vi "TreeUpdate.vi"(8 "error in":errorcluster, 11 "Data input":T1) -> (0 "error out":errorcluster, 3 "Data output":T1)   [LabVIEW 2017]
doc: "<B>This VI is used for updating tree item with Caps properties.</B>"
uses:
  API/Tree/SLSC Tree Control.lvlib
  Ctrl/Property.ctl
  Ctrl/PhysicalChannel.ctl
  Ctrl/Bitfield.ctl
  Ctrl/Register.ctl
  Ctrl/ScaleType.ctl
  Ctrl/Scale.ctl
  Ctrl/EnumValue.ctl
  Ctrl/Enum.ctl
  Ctrl/Caps.ctl
  Ctrl/Data.ctl
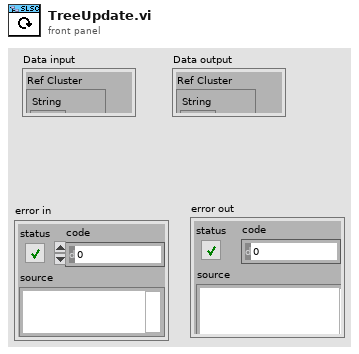
[diagram p1: front panel]
types:
  T1 = typedef "Data.ctl" = cluster{"Ref Cluster":cluster{"String":refnum<vi>, "U8":refnum<vi>, "I8":refnum<vi>, "U32":refnum<vi>, "I32":refnum<vi>, "U64":refnum<vi>, "I64":refnum<vi>, "Ring":refnum<vi>, "DBL":refnum<vi>, "Add":refnum<vi>, "Remove":refnum<vi>, "Property tree":refnum<vi>, "confirm":refnum<vi>}, "JSON Text":string, "Original JSON Text":string, "Caps":T2, "SLSC Output Tree":cluster{"Left Cell String":string, "Child Text":string[], "Child Tag":string, "Item Indent":i32, "Child Only?":bool, "Glyph Index":i32, "offline value":variant}[], "Ref Index and Control Type":cluster{"index":i32, "Datatype":string}, "Selected Type and name":cluster{"Selected Type":enum16{"Property", "Physical Channel", "Other"}, "Selected Property Name":string}, "Update whole Tree?":bool}
  T2 = typedef "Caps.ctl" = cluster{"properties":T3[], "physical channels":T4[], "registers":T5[], "scales":T7[], "enums":T9[], "productName":string}
  T3 = typedef "Property.ctl" = cluster{"name":string, "bitfield":string, "value":variant, "dataType":string, "min":variant, "max":variant, "scale":string, "access":string}
  T4 = typedef "PhysicalChannel.ctl" = cluster{"name":string, "properties":T3[]}
  T5 = typedef "Register.ctl" = cluster{"name":string, "address":i32, "size":i32, "bitfields":T6[], "initialValue":variant, "connectedProperties":string[]}
  T6 = typedef "Bitfield.ctl" = cluster{"name":string, "offset":i32, "size":i32, "signed":bool}
  T7 = typedef "Scale.ctl" = cluster{"name":string, "type":T8, "params":variant}
  T8 = typedef "ScaleType.ctl" = enum16{"NoScale", "Table", "Polynomial", "Linear"}
  T9 = typedef "Enum.ctl" = cluster{"name":string, "values":T10[]}
  T10 = typedef "EnumValue.ctl" = cluster{"name":string, "value":i32}
  T11 = cluster{"name":string, "string enums":string, "values":T10[]}[]
  T12 = cluster{"Left Cell String":string, "Child Text":string[], "Child Tag":string, "Item Indent":i32, "Child Only?":bool, "Glyph Index":i32, "offline value":variant}[]
  T13 = cluster{"Left Cell String":string, "Child Text":string[], "Child Tag":string, "Item Indent":i32, "Child Only?":bool, "Glyph Index":i32, "offline value":variant}
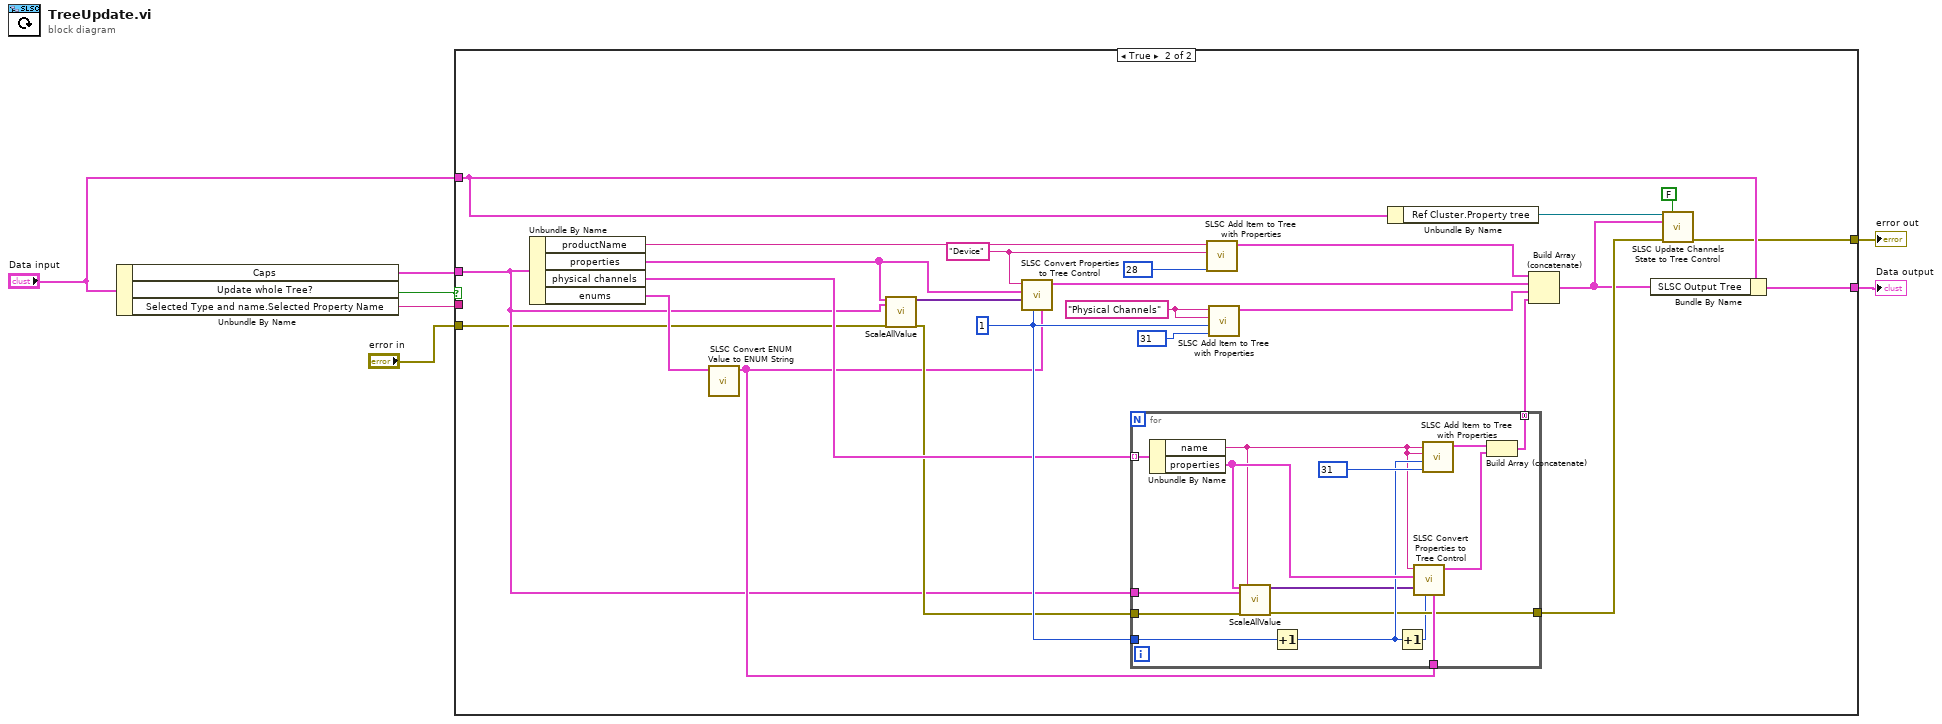
[diagram p0: block diagram]
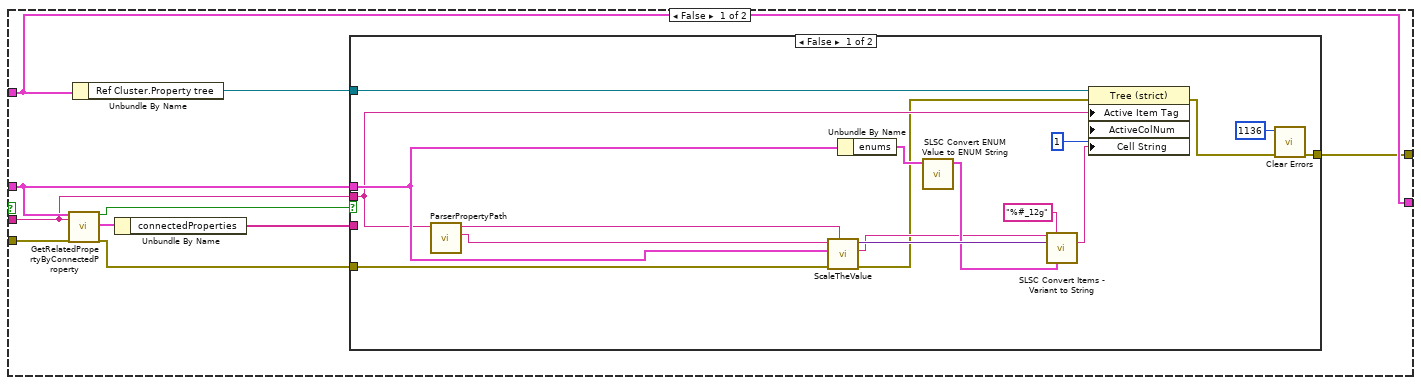
[diagram p2: hidden frame]
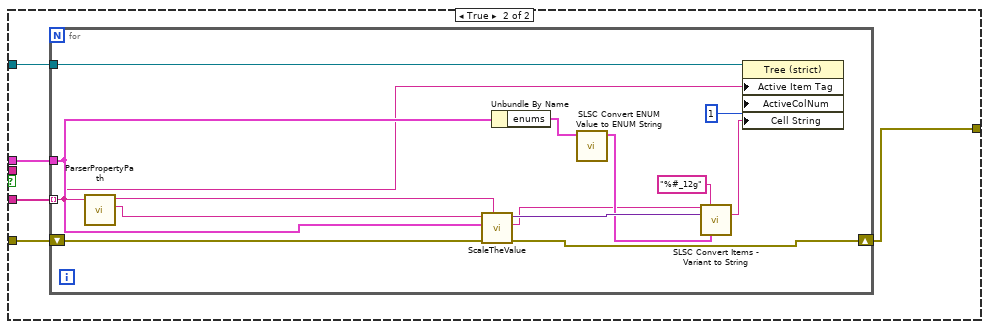
[diagram p3: hidden frame]
diagram:
  n1 = Unbundle By Name("Data input") -> ("Caps"=w6:T2, "Update whole Tree?"=w2:bool, "Selected Type and name.Selected Property Name"=w1:string)
  n2 = case shown="True" w2 {
    tunnel: [w12 w78] -> w7
    tunnel: w6 -> [w13 w57]
    tunnel: "Data input" -> [w12 w56]
    tunnel: [w10 w55] -> w4
    tunnel: w1 -> [w8 _]
    tunnel: "error in" -> [w16 w54]
    frame False {
      n3 = call "GetRelatedPropertyByConnectedProperty.vi"("Caps"=w13, "PropertyName"=w8, "error in (no error)"=w16) -> ("Find?"=w9:bool, "The Register"=w17:T5, "error out"=w11:errorcluster)  [unwired: 13 in, 1 out]
      n4 = Unbundle By Name(w12) -> ("Ref Cluster.Property tree"=w14:refnum<vi>)
      n5 = Unbundle By Name(w17) -> ("connectedProperties"=w15:string[])
      n6 = case shown="False" w9 {
        tunnel: w15 -> [_ w39]
        tunnel: w14 -> [w34 w38]
        tunnel: w13 -> [w33 w37]
        tunnel: w11 -> [w23 w36]
        tunnel: [w19 w35] -> w10
        tunnel: w8 -> [w22 _]
        frame False {
          n7 = call "ParserPropertyPath.vi"("property"=w22) -> ("name"=w29:string, "pyhsical channel"=w31:string)  [unwired: 7 in]
          n8 = call "ScaleTheValue.vi"("physical channel"=w31, "error in (no error)"=w23, "Caps"=w33, "property"=w29) -> ("error out"=w21:errorcluster, "dataType"=w24:string, "offline value"=w27:variant)  [unwired: 5 in]
          n9 = Unbundle By Name(w33) -> ("enums"=w30:T9[])
          n10 = call "SLSC Convert ENUM Value to ENUM String.vi"("enums"=w30) -> ("string enums"=w26:T11)  [unwired: 10 in]
          n11 = call "SLSC Convert Items - Variant to String.vi"("dataType"=w24, "format string"="%#_12g", "value"=w27, "string enums"=w26) -> ("string offline data value"=w25:string)  [unwired: 7 in, 4 out]
          n12 = property class="Tree (strict)"(reference=w34, error in=w21, "Active Item Tag"=w22, "ActiveColNum"=1 ("Active Cell:Active Column Number"), "Cell String"=w25) -> (error out=w20:errorcluster)  [unwired: 1 out]
          n13 = call <vilib>:"Clear Errors.vi"("error in (no error)"=w20, "specific error code to clear (0: all)"=1136) -> ("error out"=w19:errorcluster)  [unwired: 4 in, 1 out]
        }
        frame True {
          n14 = for {
            tunnel: w39 -> [w40] mode=indexing
            tunnel: w38 -> [w53]
            tunnel: w37 -> [w50]
            shift-right: [w42] -> w35
            shift-left: w36 -> [w43]
            n15 = call "ParserPropertyPath.vi"("property"=w40) -> ("name"=w48:string, "pyhsical channel"=w51:string)  [unwired: 7 in]
            n16 = call "ScaleTheValue.vi"("physical channel"=w51, "error in (no error)"=w43, "Caps"=w50, "property"=w48) -> ("error out"=w42:errorcluster, "dataType"=w41:string, "offline value"=w46:variant)  [unwired: 5 in]
            n17 = Unbundle By Name(w50) -> ("enums"=w49:T9[])
            n18 = call "SLSC Convert ENUM Value to ENUM String.vi"("enums"=w49) -> ("string enums"=w45:T11)  [unwired: 10 in]
            n19 = call "SLSC Convert Items - Variant to String.vi"("dataType"=w41, "format string"="%#_12g", "value"=w46, "string enums"=w45) -> ("string offline data value"=w44:string)  [unwired: 7 in, 4 out]
            n20 = property class="Tree (strict)"(reference=w53, "Active Item Tag"=w40, "ActiveColNum"=1 ("Active Cell:Active Column Number"), "Cell String"=w44) -> ()  [unwired: 1 in, 2 out]
          }
        }
      }
    }
    frame True {
      w72 = 1
      w74 = "Physical Channels"
      w76 = "Device"
      n21 = Unbundle By Name(w57) -> ("productName"=w68:string, "properties"=w70:T3[], "physical channels"=w67:T4[], "enums"=w71:T9[])
      n22 = call "SLSC Convert ENUM Value to ENUM String.vi"("enums"=w71) -> ("string enums"=w59:T11)  [unwired: 10 in]
      n23 = call "ScaleAllValue.vi"("properties"=w70, "Caps"=w57, "error in (no error)"=w54) -> ("Init Value"=w69:variant[], "error out"=w60:errorcluster)  [unwired: 15 in]
      n24 = call "SLSC Convert Properties to Tree Control.vi"("string enums"=w59, "Item Indent"=w72, "Init Values"=w69, "properties"=w70, "Child Tag"=w76) -> ("Tree Items"=w63:T12)  [unwired: 6 in]
      n25 = for {
        tunnel: w67 -> [w93] mode=indexing
        tunnel: w60 -> [w92]
        tunnel: w59 -> [w87]
        tunnel: w72 -> [w86]
        tunnel: [w84] -> w66 mode=concatenating
        tunnel: [w83] -> w61
        tunnel: w57 -> [w82]
        n26 = Unbundle By Name(w93) -> ("name"=w81:string, "properties"=w90:T3[])
        n27 = call "ScaleAllValue.vi"("properties"=w90, "Caps"=w82, "error in (no error)"=w92, "physical channel"=w81) -> ("Init Value"=w80:variant[], "error out"=w83:errorcluster)  [unwired: 14 in]
        n28 = Increment(x=w86) -> (x+1=w85:i32)
        n29 = Increment(x=w85) -> (x+1=w79:i32)
        n30 = call "SLSC Convert Properties to Tree Control.vi"("string enums"=w87, "Item Indent"=w79, "Init Values"=w80, "properties"=w90, "Child Tag"=w81) -> ("Tree Items"=w88:T12)  [unwired: 6 in]
        n31 = call "SLSC Add Item to Tree with Properties.vi"("Glyph Index"=31, "Item indent"=w85, "Child Tag"=w81, "Left Cell String"=w81) -> ("Item"=w89:T13)  [unwired: 7 in]
        n32 = Build Array (concatenate)(w89, w88) -> (w84:T12)
      }
      n33 = call "SLSC Add Item to Tree with Properties.vi"("Glyph Index"=28, "Child Tag"=w76, "Left Cell String"=w68) -> ("Item"=w64:T13)  [unwired: 8 in]
      n34 = call "SLSC Add Item to Tree with Properties.vi"("Glyph Index"=31, "Item indent"=w72, "Child Tag"=w74, "Left Cell String"=w74) -> ("Item"=w65:T13)  [unwired: 7 in]
      n35 = Unbundle By Name(w56) -> ("Ref Cluster.Property tree"=w62:refnum<vi>)
      n36 = Build Array (concatenate)(w64, w63, w65, w66) -> (w58:T12)
      n37 = Bundle By Name(cluster=w56, "SLSC Output Tree"=w58) -> (w78:T1)
      n38 = call "SLSC Update Channels State to Tree Control.vi"("Property tree"=w62, "Update Only?"=FALSE, "SLSC Output Tree"=w58, "error in (no error)"=w61) -> ("error out"=w55:errorcluster)  [unwired: 11 in]
    }
  }
  "Data output" <- w7
  "error out" <- w4
